vi "Credit update.vi"(8 "error in (no error)":errorcluster, 10 "Creditp":dbl, 11 "UI Actor in":refnum<class "UI Actor.lvclass">) -> (0 "error out":errorcluster, 3 "UI Actor out":refnum<class "UI Actor.lvclass">)   [LabVIEW 2020, in "UI Actor.lvlib" / "UI Actor.lvclass"]
uses:
  UI Actor.lvclass
  UI Actor.lvclass/UI Actor.ctl
  MSG Messages/Update msg Msg/Update msg Msg.lvclass/Update msg Msg.ctl
  <vilib>/ActorFramework/Message Enqueuer/Message Enqueuer.lvclass/Message Enqueuer.ctl
  <vilib>/ActorFramework/Message Enqueuer/Enqueue.vi
  MSG Messages/Update msg Msg/Update msg Msg.lvclass
  C:/Program Files/National Instruments/LabVIEW 2020/vi.lib/ActorFramework/Message/Message.lvclass
  <vilib>/ActorFramework/Message Priority Queue/Priority Enqueue.vi
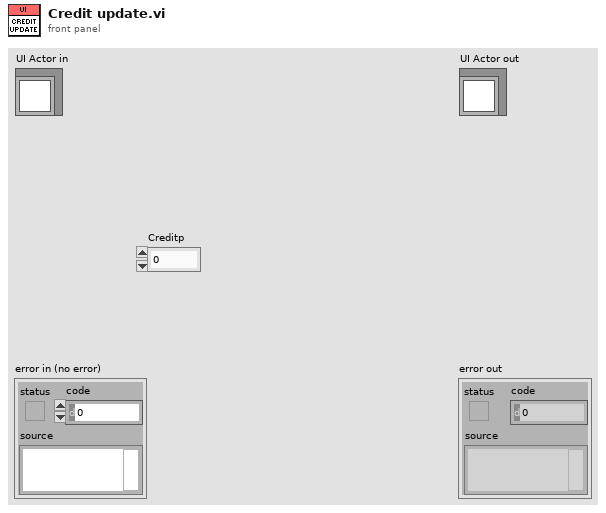
[diagram p1: front panel]
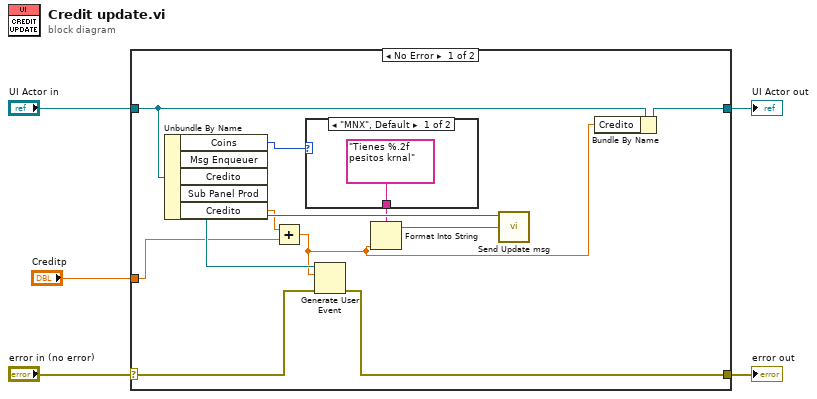
[diagram p0: block diagram]
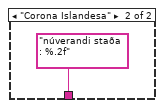
[diagram p2: hidden frame]
diagram:
  n1 = case shown="No Error" "error in (no error)" {
    selector: "error in (no error)" -> [w15 w21]
    tunnel: [w14 w21] -> w4
    tunnel: [w9 w20] -> w2
    tunnel: "UI Actor in" -> [w17 w20]
    tunnel: "Creditp" -> [w7 _]
    frame No Error {
      n2 = Unbundle By Name(w17) -> ("Coins"=w10:enum16{"MNX", "Corona Islandesa"}, "Msg Enqueuer"=w13:refnum<class "Message Enqueuer.lvclass">, "Credito"=w16:refnum<user-event>, "Credito"=w8:dbl)  [unwired: 1 out]
      n3 = Add(x=w8, y=w7) -> (x+y=w6:dbl)
      n4 = case shown="\"MNX\", Default" w10 {
        tunnel: ["Tienes %.2f pesitos krnal" ("format string") "núverandi staða : %.2f" ("format string")] -> w11
        frame "MNX", Default {
        }
        frame "Corona Islandesa" {
        }
      }
      n5 = Generate User Event(user event=w16, event data cluster=w6, error in=w15) -> (error out=w14:errorcluster)  [unwired: 1 in, 1 out]
      n6 = Format Into String(format string=w11, w6) -> (resulting string=w12:string)  [unwired: 2 in, 1 out]
      n7 = call "Send Update msg.vi"("Update msg"=w12, "Message Enqueuer"=w13) -> ()  [unwired: 8 in, 2 out]
      n8 = Bundle By Name(cluster=w17, "Credito"=w6) -> (w9:refnum<class "UI Actor.lvclass">)
    }
    frame Error {
    }
  }
  "error out" <- w4
  "UI Actor out" <- w2
